vi "Get Gabor Window Info.vi"(8 "error in (no error)":errorcluster, 11 "RefNum in":T1) -> (0 "error out":errorcluster, 1 "synthesis window":cluster{"g[i]":dbl[], "dM":i32, "length":i32} {"g[i]" format="%.2f"}, 2 "analysis window":cluster{"gamma[i]":dbl[], "dM":i32, "N":i32} {"gamma[i]" format="%.2f"}, 3 "RefNum out":T1)   [LabVIEW 2017, in "SoundVib_Gabor.lvlib"]
doc: "Retrieves information about <B>analysis window</B>, which you use in Gabor transform, and <B>synthesis window</B>, which you use in Gabor expansion. The Easy Gabor Transform VI generates <B>analysis window</B> and <B>synthesis window</B> and stores them in the data block referenced by <B>RefNum in</B>."
uses:
  <vilib>/addons/Sound and Vibration/Order Analysis/Gabor Order Tracking/SoundVib_Gabor.lvlib
  <vilib>/addons/Sound and Vibration/Order Analysis/Ref Gabor Order Tracking/GT RefNum.ctl
  <resource>/sndvib.dll
panel:
  # "Get Gabor Windows Info"
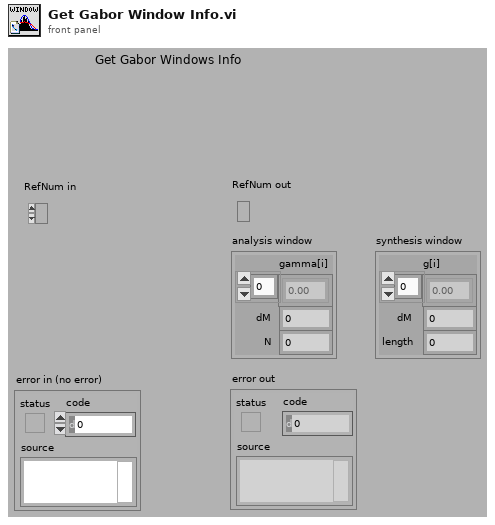
[diagram p1: front panel]
types:
  T1 = typedef "SoundVib_Gabor.lvlib/GT RefNum.ctl" = refnum<k1>
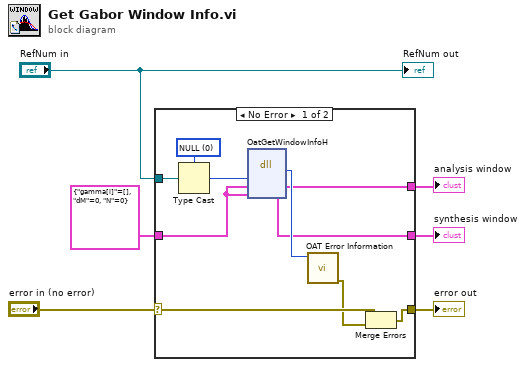
[diagram p0: block diagram]
diagram:
  n1 = case shown="No Error" "error in (no error)" {
    selector: "error in (no error)" -> [w9 w18]
    tunnel: [w7 w18] -> w6
    tunnel: "RefNum in" -> [w11 _]
    tunnel: [w13 w17] -> w3
    tunnel: [w12 w17] -> w2
    tunnel: cluster{"gamma[i]":dbl[], "dM":i32, "N":i32} {"gamma[i]"=[], "dM"=0, "N"=0} ("Analysis Window Info.") -> [w10 w17]
    frame No Error {
      w14 = u32 0 items=["NULL"]
      n2 = Type Cast(type=w14, x=w11) -> (*(type *) &x=w15:u32)
      n3 = dll-call lib="C:/Program Files (x86)/National Instruments/LabVIEW 2017/resource/sndvib.*" fn="OatGetWindowInfoH"("Ref In"=w15, "Analysis Window"=w10, "Synthesis Window"=w10) -> ("return type"=w16:i32, "Analysis Window"=w13:cluster{"gamma[i]":dbl[], "dM":i32, "N":i32}, "Synthesis Window"=w12:cluster{"gamma[i]":dbl[], "dM":i32, "N":i32})  [unwired: 4 in, 2 out]
      n4 = call <vilib>:"OAT Error Information.vi"("error code"=w16) -> ("error out"=w8:errorcluster)  [unwired: 6 in]
      n5 = Merge Errors(w9, w8) -> (w7:errorcluster)
    }
    frame Error {
    }
  }
  "error out" <- w6
  "synthesis window" <- w2
  "analysis window" <- w3
  "RefNum out" <- "RefNum in"
